vi "runFirstState.vi"(6 "Fault?":bool, 7 "Ready":bool, 8 "error in (no error)":errorcluster, 9 "Actuators in":T1, 10 "State in":T2, 11 "FullRun in":refnum<class "FullRun.lvclass">) -> (0 "error out":errorcluster, 1 "Actuators out":T1, 2 "State out":T2, 3 "FullRun out":refnum<class "FullRun.lvclass">)   [LabVIEW 2018, in "ControlLibrary.lvlib" / "FullRun.lvclass"]
uses:
  FullRun.lvclass
  TypeDef_ControlState.ctl
  TypeDef_DigitalOuts.ctl
  RunTypeClass/RunType.lvclass
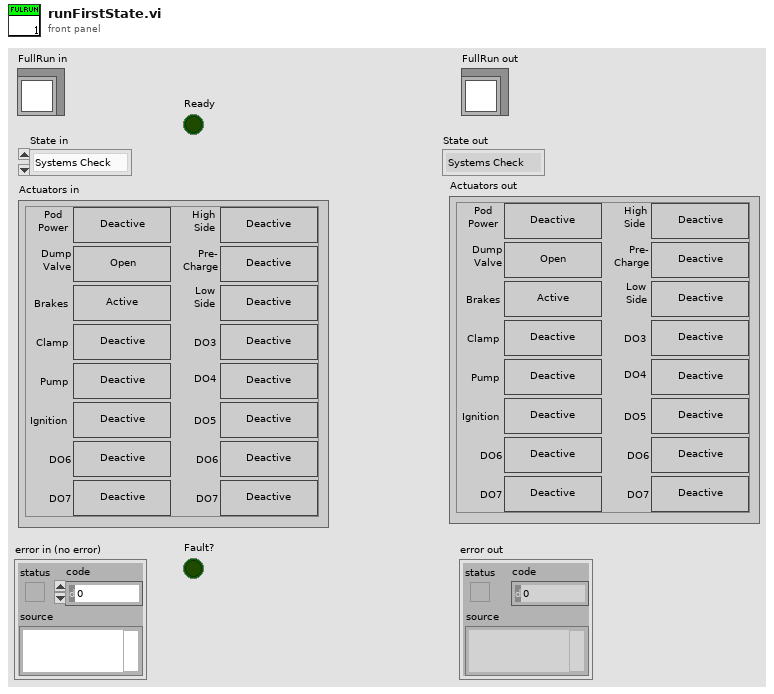
[diagram p1: front panel]
types:
  T1 = typedef "TypeDef_DigitalOuts.ctl" = cluster{"Pod Power":bool, "Dump Valve":bool, "Brakes":bool, "Clamp":bool, "Pump":bool, "Ignition":bool, "DO6":bool, "DO7":bool, "HighSide":bool, "Precharge":bool, "LowSide":bool, "DO3":bool, "DO4":bool, "DO5":bool, "DO62":bool, "DO72":bool}
  T2 = typedef "TypeDef_ControlState.ctl" = enum16{"Systems Check", "Idle", "Ready", "Pushing", "Coast", "Braking", "Fault", "Shutdown", "Service", "Precharge", "Blank"}
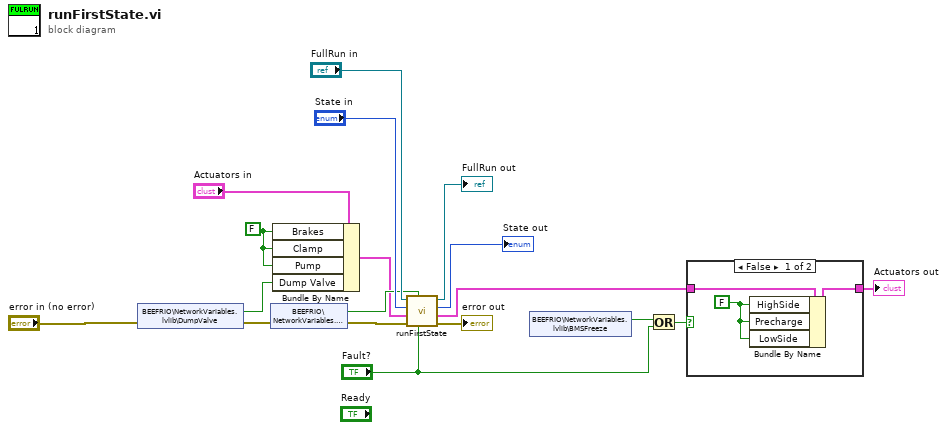
[diagram p0: block diagram]
diagram:
  w8 = FALSE ("Brakes")
  n1 = shared-variable "BEEFRIO\\NetworkVariables.lvlib\\DumpValve"(error in="error in (no error)") -> (w9:bool, error out=w14:errorcluster)
  n2 = shared-variable "BEEFRIO\\NetworkVariables.lvlib\\Ready"(error in=w14) -> (w13:bool, error out=w11:errorcluster)
  n3 = Bundle By Name(cluster="Actuators in", "Brakes"=w8, "Clamp"=w8, "Pump"=w8, "Dump Valve"=w9) -> (w12:T1)
  n4 = call-parent "runFirstState.vi"("Fault?"="Fault?", "Ready"=w13, "error in (no error)"=w11, "Actuators in"=w12, "State in"="State in", "RunType in"="FullRun in") -> ("error out"=→"error out":errorcluster, "Actuators out"=w2:T1, "State out"=→"State out":T2, "RunType out"=→"FullRun out":refnum<class "FullRun.lvclass">)  [unwired: 2 in]
  n5 = shared-variable "BEEFRIO\\NetworkVariables.lvlib\\BMSFreeze"() -> (w4:bool)  [unwired: 1 in, 1 out]
  n6 = Or(x=w4, y="Fault?") -> (x .or. y?=w3:bool)
  n7 = case shown="False" w3 {
    tunnel: w2 -> [w20 w22]
    tunnel: [w21 w22] -> w1
    frame False {
      w19 = FALSE ("HighSide")
      n8 = Bundle By Name(cluster=w20, "HighSide"=w19, "Precharge"=w19, "LowSide"=w19) -> (w21:T1)
    }
    frame True {
    }
  }
  "Actuators out" <- w1
